vi "ziModSetValueBinaryArray.vi"(8 "Error In":errorcluster, 9 "Values":string[](array[string]), 10 "Paths":string[](array[string]), 11 "ModHandle In":T1 {"ModHandle" format="0x%08x"; "Conn" format="0x%08x"}) -> (0 "Error Out":errorcluster, 3 "ModHandle Out":T1 {"ModHandle" format="0x%08x"; "Conn" format="0x%08x"})   [LabVIEW 2009, in "Zurich Instruments LabOne.lvlib"]
doc: "This vi sets values of the specified <b>module </b> nodes in <b>Path</b> to <b>Value</b>., e.g sweep/endless"
uses:
  <instrlib>/Zurich Instruments LabOne/Zurich Instruments LabOne.lvlib
  <instrlib>/Zurich Instruments LabOne/Public/Modules/ziTypeModHandle.ctl
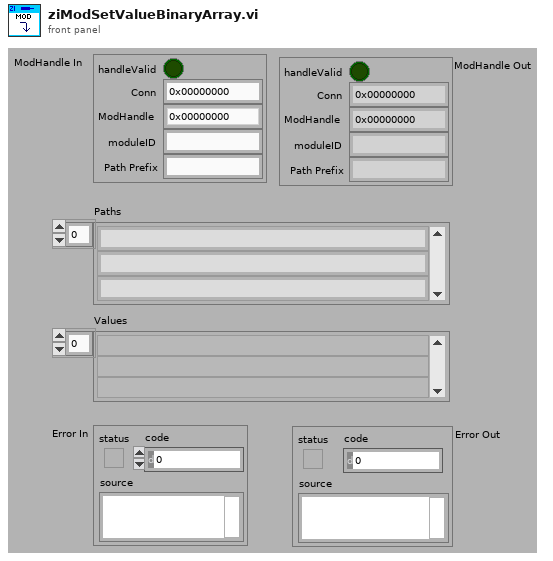
[diagram p1: front panel]
types:
  T1 = typedef "Zurich Instruments LabOne.lvlib/ziTypeModHandle.ctl" = cluster{"handleValid":bool, "Conn":u64, "ModHandle":u64, "moduleID":string, "Path Prefix":string}
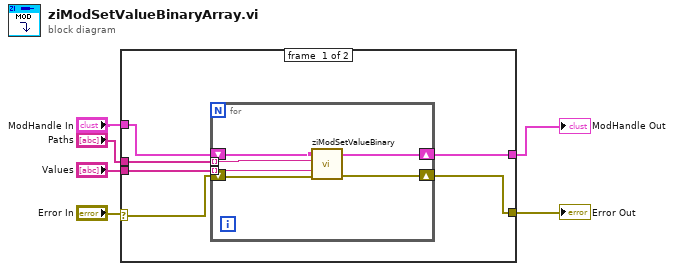
[diagram p0: block diagram]
diagram:
  n1 = case shown="No Error" "Error In" {
    selector: "Error In" -> [w9 w20]
    tunnel: [w10 w20] -> w6
    tunnel: "ModHandle In" -> [w12 w19]
    tunnel: [w11 w19] -> w3
    tunnel: "Paths" -> [w8 _]
    tunnel: "Values" -> [w7 _]
    frame #0 {
      n2 = for {
        tunnel: w8 -> [w18] mode=indexing
        shift-right: [w16] -> w10
        shift-left: w9 -> [w17]
        shift-right: [w15] -> w11
        shift-left: w12 -> [w14]
        tunnel: w7 -> [w13] mode=indexing
        n3 = call <instrlib>:"ziModSetValueBinary.vi"("Error In"=w17, "Data"=w13, "Path"=w18, "ModHandle In"=w14) -> ("Error Out"=w16:errorcluster, "ModHandle Out"=w15:T1)  [unwired: 6 in]
      }
    }
    frame #1 {
    }
  }
  "Error Out" <- w6
  "ModHandle Out" <- w3
